vi "Write Form path.vi"(8 "error in (no error)":errorcluster, 10 "Form path":path, 11 "Form Configuration in":refnum<class "Form Configuration.lvclass">) -> (0 "error out":errorcluster, 3 "Form Configuration out":refnum<class "Form Configuration.lvclass">)   [LabVIEW 2020, in "Form Configuration.lvlib" / "Form Configuration.lvclass"]
uses:
  Form Configuration.lvclass
  Form Configuration.lvclass/Form Configuration.ctl
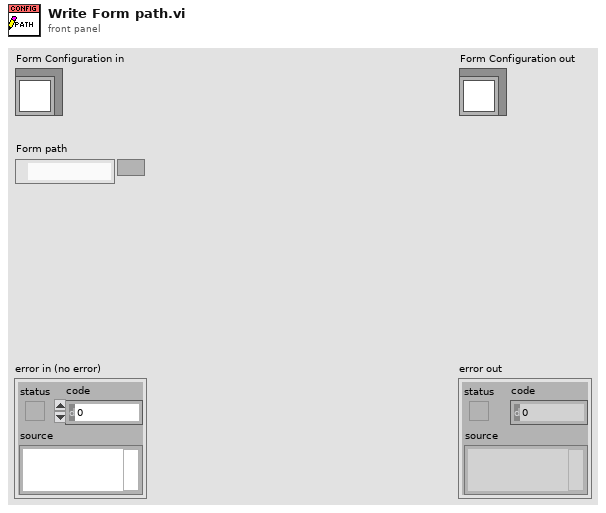
[diagram p1: front panel]
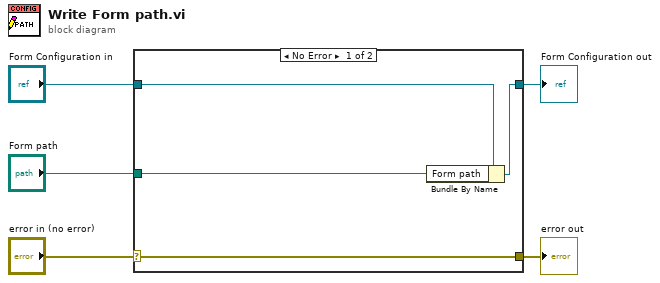
[diagram p0: block diagram]
diagram:
  n1 = case shown="No Error" "error in (no error)" {
    selector: "error in (no error)" -> [w9 w10]
    tunnel: [w9 w10] -> w4
    tunnel: [w7 w11] -> w2
    tunnel: "Form Configuration in" -> [w8 w11]
    tunnel: "Form path" -> [w6 _]
    frame No Error {
      n2 = Bundle By Name(cluster=w8, "Form path"=w6) -> (w7:refnum<class "Form Configuration.lvclass">)
    }
    frame Error {
    }
  }
  "error out" <- w4
  "Form Configuration out" <- w2
